vi "error_codes_array.vi"(8 "?":errorcluster, 9 "Boolean":bool, 10 "String":string) -> (0 "?":errorcluster={"status"=FALSE, "code"=1073676294, "source"="VISA Read in query.vi->get_laser_status.vi->vitesse.vi"}, 2 "Array":i32[](array[numeric]))   [LabVIEW 2013]
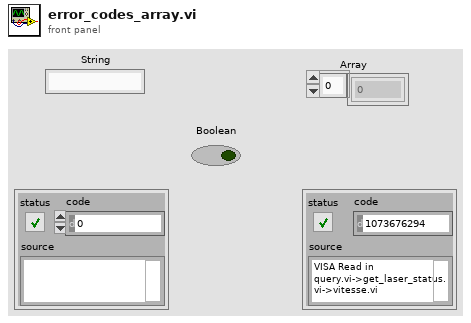
[diagram p1: front panel]
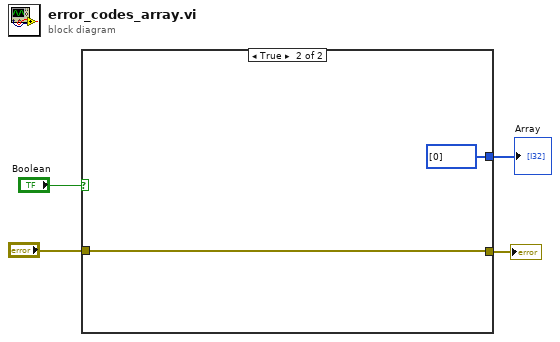
[diagram p0: block diagram]
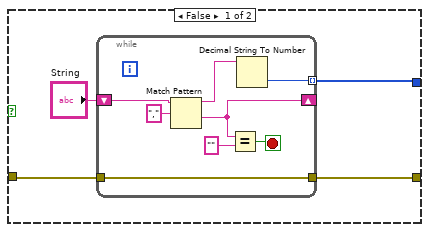
[diagram p2: hidden frame]
diagram:
  n1 = case shown="True" "Boolean" {
    tunnel: [w7 i32[] [0]] -> w3
    tunnel: [w6 w18] -> w2
    tunnel: "?" -> [w5 w18]
    frame False {
      n2 = while {
        shift-right: [w12] -> _
        shift-left: "String" -> [w15]
        tunnel: [w10] -> w7 mode=indexing
        tunnel: w5 -> [w9]
        tunnel: [w9] -> w6
        stop <- w14 stop-if-true
        n3 = Match Pattern(string=w15, regular expression=",") -> (before substring=w11:string, after substring=w12:string)  [unwired: 1 in, 2 out]
        n4 = Equal?(x=w12, y="") -> (x = y?=w14:bool)
        n5 = Decimal String To Number(string=w11) -> (number=w10:i32)  [unwired: 2 in, 1 out]
      }
    }
    frame True {
    }
  }
  "Array" <- w3
  "?" <- w2
